vi "Set Run Icon Editor from Source.vi"   [LabVIEW 2020]
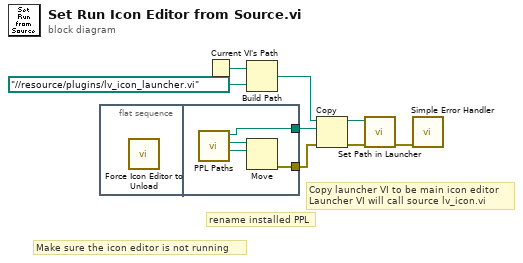
[diagram p0: block diagram]
diagram:
  # "Copy launcher VI to be main icon editor\nLauncher VI will call source lv_icon.vi"
  # "rename installed PPL"
  # "Make sure the icon editor is not running"
  n1 = flat-sequence {
    tunnel: [w12] -> w8
    tunnel: [w9] -> w3
    frame #0 {
      n2 = call "Force Icon Editor to Unload.vi"() -> ()  [unwired: 12 in]
    }
    frame #1 {
      n3 = call "PPL Paths.vi"() -> ("Renamed PPL Path"=w11:path, "PPL Path"=w10:path, "lv_icon Path"=w9:path)  [unwired: 9 in]
      n4 = Move(source path=w10, 10:w11) -> (error out=w12:errorcluster)  [unwired: 3 in, 2 out]
    }
  }
  n5 = Current VI's Path() -> (path=w5:path)
  n6 = Build Path(base path=w5, name or relative path=path "../../resource/plugins/lv_icon_launcher.vi") -> (appended path=w2:path)
  n7 = Copy(8:w8, 10:w3, 11:w2) -> (0:w7:errorcluster, 3:w1:path)  [unwired: 2 in, 1 out]
  n8 = call "Set Path in Launcher.vi"("error in"=w7, "launcher path"=w1) -> ("error out"=w6:errorcluster)  [unwired: 9 in]
  n9 = call <vilib>:"Simple Error Handler.vi"("error in (no error)"=w6) -> ()  [unwired: 4 in, 5 out]
